vi "stepper controller -- BLM.vi"(7 "stepper driver action":T2, 8 "set":dbl format="%#_13g", 9 "stepper motor state":T1) -> (1 "stepper motor state OUT":T1)   [LabVIEW 2018]
uses:
  IMS Stepper Controller/stepper motor state.ctl
  IMS Stepper Controller/stepper motor action.ctl
  stack action -- control.ctl
  internal stepper driver state -- BLM.ctl
panel:
  in  "VISA session":refnum<visa-resource-name>="GPIB0::25::INSTR"
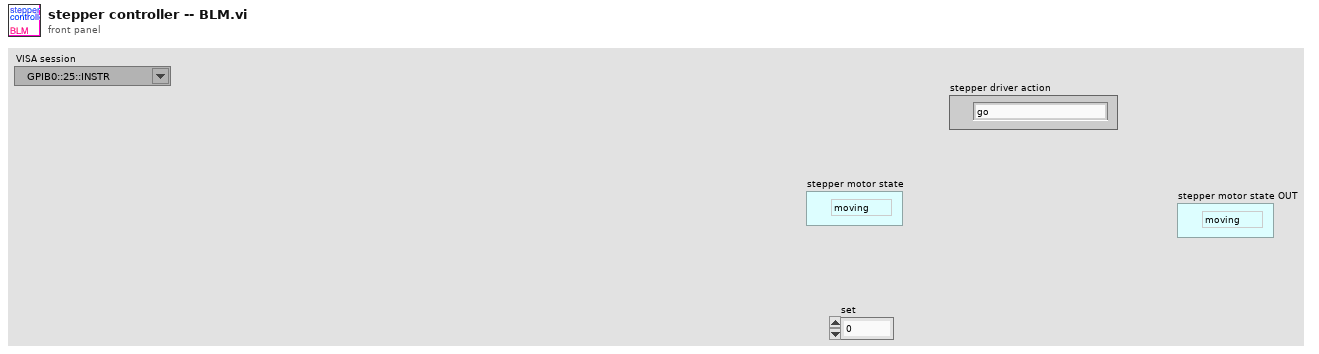
[diagram p1: front panel]
types:
  T1 = typedef "stepper motor state.ctl" = enum16{"moving", "stopped"}
  T2 = typedef "stepper motor action.ctl" = enum16{"go", "stop", "check", "init", "sync", "set", "set speed", "void"}
  T3 = typedef "stack action -- control.ctl" = enum16{"push", "pop", "check", "init"}
  T4 = typedef "internal stepper driver state -- BLM.ctl" = cluster{"initialized?":bool, "VISA session":refnum<visa-resource-name>, "stepper motor state":T1}
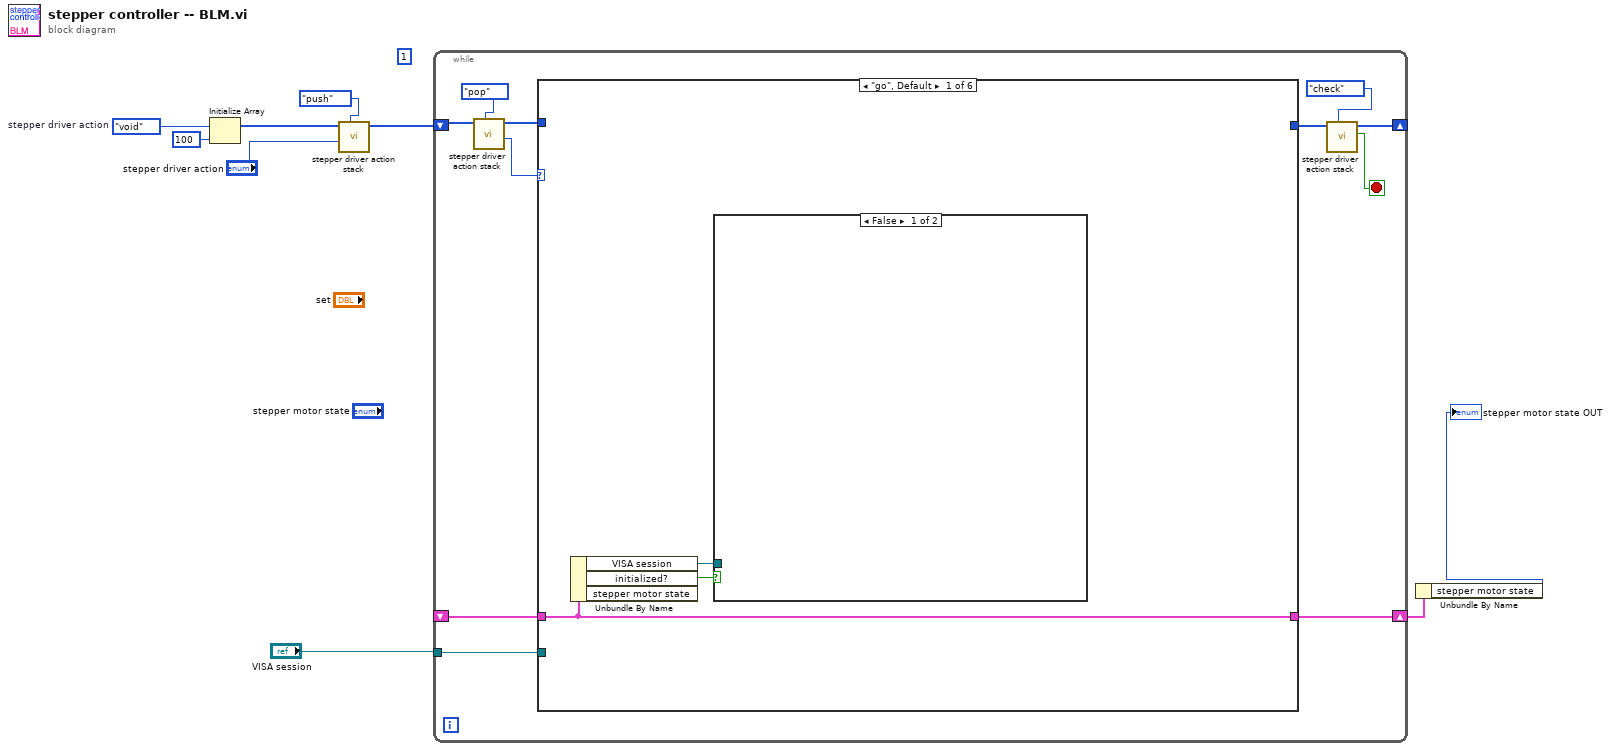
[diagram p0: block diagram]
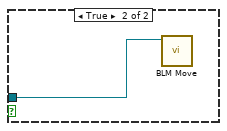
[diagram p2: hidden frame]
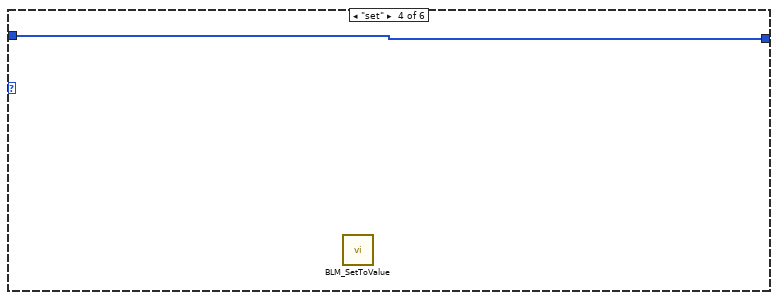
[diagram p5: hidden frame]
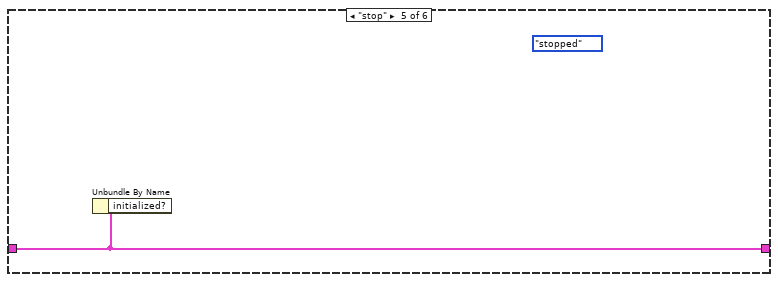
[diagram p6: hidden frame]
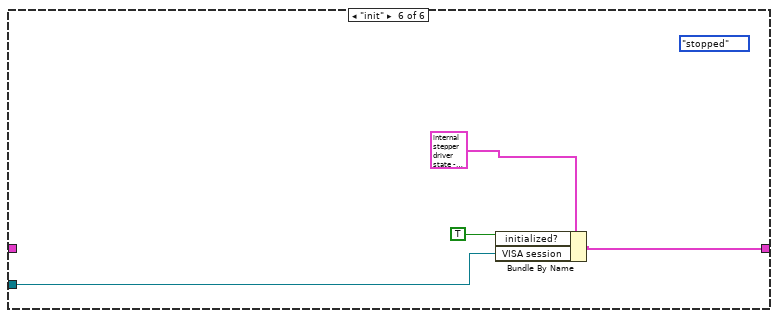
[diagram p7: hidden frame]
diagram:
  w8 = stepper_motor_action."void"  # stepper driver action
  (unwired) 1
  n1 = Initialize Array(w8, 100 ("dimension size")) -> (w6:T2[])
  n2 = call "stepper driver action stack.vi"("stack action"=stack_action_--_control."push", "stepper driver action IN"="stepper driver action", "stack IN"=w6) -> ("command stack OUT"=w3:T2[])  [unwired: 6 in, 2 out]
  n3 = while {
    shift-right: [w20] -> w2
    shift-left: _ -> [w19]
    tunnel: "VISA session" -> [w18]
    shift-right: [w12] -> _
    shift-left: w3 -> [w16]
    stop <- w10 stop-if-true
    n4 = call "stepper driver action stack.vi"("stack action"=stack_action_--_control."pop", "stack IN"=w16) -> ("stepper driver action  OUT"=w15:T2, "command stack OUT"=w14:T2[])  [unwired: 7 in, 1 out]
    n5 = case shown="\"go\", Default" w15 {
      tunnel: [w23 _ _ _ w26 w30] -> w20
      tunnel: w19 -> [w23 _ _ _ w26 _]
      tunnel: w18 -> [_ _ _ _ _ w28]
      tunnel: [_ _ _ w25 _ _] -> w13
      tunnel: w14 -> [_ _ _ w25 _ _]
      frame "go", Default {
        n6 = Unbundle By Name(w23) -> ("VISA session"=w21:refnum<visa-resource-name>, "initialized?"=w22:bool)  [unwired: 1 out]
        n7 = case shown="False" w22 {
          tunnel: w21 -> [_ w24]
          frame False {
          }
          frame True {
            n8 = call "BLM Move.vi"("Port Address"=w24) -> ()  [unwired: 5 in, 1 out]
          }
        }
      }
      frame "check" {
      }
      frame "sync" {
      }
      frame "set" {
        n9 = call "BLM_SetToValue.vi"() -> ()  [unwired: 4 in, 1 out]
      }
      frame "stop" {
        (unwired) stepper_motor_state."stopped" ("stepper motor state")
        n10 = Unbundle By Name(w26) -> ()  [unwired: 1 out]
      }
      frame "init" {
        (unwired) stepper_motor_state."stopped" ("stepper motor state")
        n11 = Bundle By Name(cluster=T4 {"initialized?"=TRUE, "VISA session"="GPIB0::25::INSTR", "stepper motor state"=enum."moving"} ("internal stepper driver state BLM"), "initialized?"=TRUE, "VISA session"=w28) -> (w30:T4)
      }
    }
    n12 = call "stepper driver action stack.vi"("stack action"=stack_action_--_control."check", "stack IN"=w13) -> ("stack is empty ?"=w10:bool, "command stack OUT"=w12:T2[])  [unwired: 7 in, 1 out]
  }
  n13 = Unbundle By Name(w2) -> ("stepper motor state"=→"stepper motor state OUT":T1)
